vi "TH_Ini_Parameters.vi"() -> ()   [LabVIEW 2020]
panel:
  out "DeviceId3":string
  out "DeviceId2":string
  out "DeviceId1":string
  out "Bladmögel":bool
  out "Port3":string
  out "Port2":string
  out "Port1":string
  out "Device3":i32
  out "Device2":i32
  out "Device1":i32
  out "Port":string
  out "SensorType":string
  # "Parameters read from the TH-Logger.ini file"
  # "NH485"
  # "HygroWin"
  # "TelldusLive"
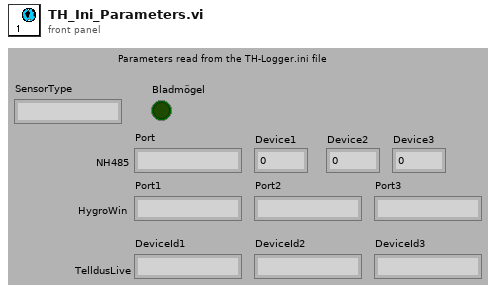
[diagram p1: front panel]
diagram:
